vi "To Scanreader XML String.vi"(8 "Use LCD?":bool, 9 "Reader":T2, 10 "Scanner 2 (second scan axis)":T1=enum."None", 11 "Scanner":T1) -> (3 "xml string":string)   [LabVIEW 2017, in "Scan Driver.lvclass"]
uses:
  Scan Driver.lvclass
  Reader List.ctl
  Scanner List.ctl
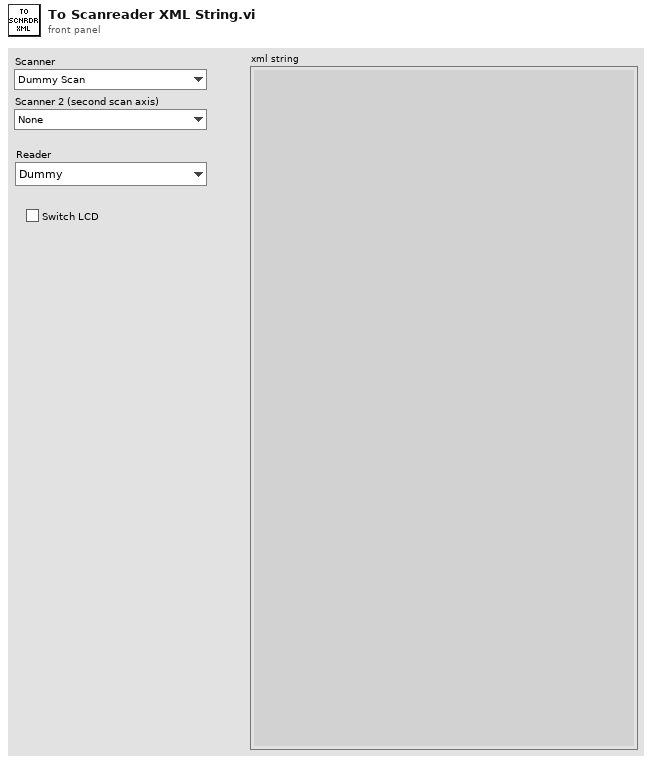
[diagram p1: front panel]
types:
  T1 = typedef "Scan Driver.lvclass/Scanner List.ctl" = enum16{"Dummy Scan", "Analog Output Scan", "Function Gen Scan", "Magna Current Scan", "Magna Voltage Scan", "Magnetic Field Lakeshore", "Magnetic Field Lakeshore Continuous", "Magnetic Field Oxford", "Magnetic Field Oxford Continuous", "Microwave Freq Scan", "Pulse Gen Basic Scan", "Pulse Gen Scan", "Translation Stage Coarse", "Translation Stage Dual", "Translation Stage Fine", "Wavelength ActiveX", "Wavelength Digikröm", "Wavelength Triax 550", "None"}
  T2 = typedef "Scan Driver.lvclass/Reader List.ctl" = enum16{"Dummy", "Cryostat Temperature", "DAQmx Analog", "Lockin SR810", "Lockin SR830", "Fluke Multimeter", "Photon Counter Reader", "Power Meter", "Temperature Control", "Two Lockins"}
  T3 = cluster{"Scanner":T1, "Scanner 2 (second scan axis)":T1, "Reader":T2, "Use LCD?":bool}
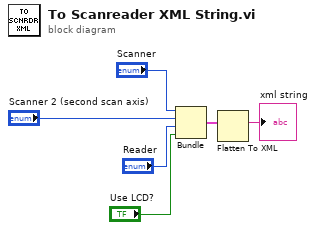
[diagram p0: block diagram]
diagram:
  n1 = Bundle("Scanner"="Scanner", "Scanner 2 (second scan axis)"="Scanner 2 (second scan axis)", "Reader"="Reader", "Use LCD?"="Use LCD?") -> (w1:T3)  [unwired: 1 in]
  n2 = Flatten To XML(anything=w1) -> (xml string=→"xml string":string)
